vi "Initialize Digital IO.vi"(8 "error in (no error)":errorcluster, 11 "DigitalIO in":refnum<class "DigitalIO.lvclass">) -> (0 "error out":errorcluster, 3 "DigitalIO out":refnum<class "DigitalIO.lvclass">)   [LabVIEW 2018, in "DigitalIO.lvlib" / "DigitalIO.lvclass"]
uses:
  DigitalIO.lvclass
  DigitalIO.lvclass/DigitalIO.ctl
  PPLs/Configuration/Configuration.lvlibp/Configuration.lvclass
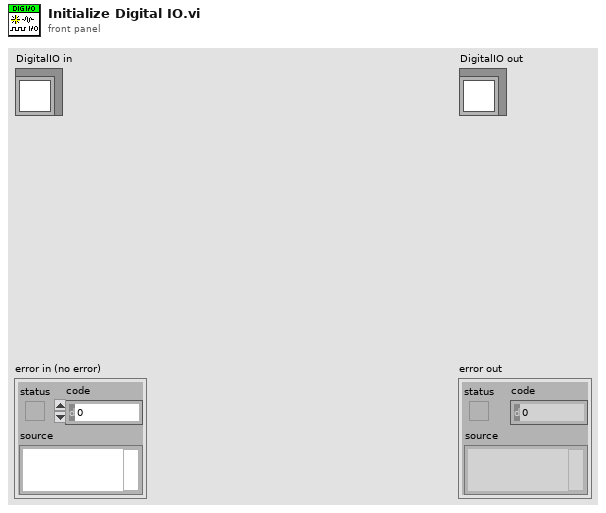
[diagram p1: front panel]
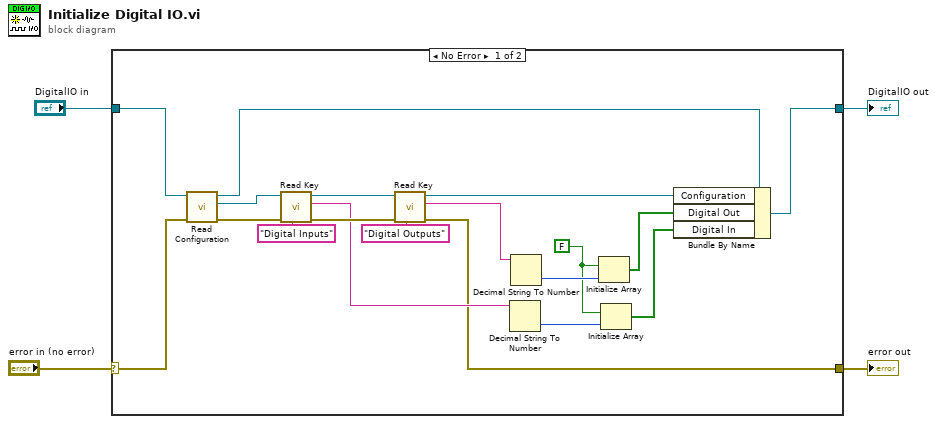
[diagram p0: block diagram]
diagram:
  n1 = case shown="No Error" "error in (no error)" {
    selector: "error in (no error)" -> [w23 w25]
    tunnel: [w5 w25] -> w1
    tunnel: [w6 w24] -> w2
    tunnel: "DigitalIO in" -> [w22 w24]
    frame No Error {
      w11 = FALSE
      n2 = call "Read Configuration.vi"("error in (no error)"=w23, "DigitalIO in"=w22) -> ("error out"=w20:errorcluster, "Configuration"=w21:refnum<class "Configuration.lvclass">, "DigitalIO out"=w10:refnum<class "DigitalIO.lvclass">)  [unwired: 7 in]
      n3 = call "Read Key.vi"("Key:"="Digital Inputs", "error in"=w20, "Configuration in"=w21) -> ("error out"=w16:errorcluster, "Value"=w15:string, "Configuration out"=w17:refnum<class "Configuration.lvclass">)  [unwired: 6 in]
      n4 = call "Read Key.vi"("Key:"="Digital Outputs", "error in"=w16, "Configuration in"=w17) -> ("error out"=w5:errorcluster, "Value"=w14:string, "Configuration out"=w9:refnum<class "Configuration.lvclass">)  [unwired: 6 in]
      n5 = Decimal String To Number(string=w15) -> (number=w12:i32)  [unwired: 2 in, 1 out]
      n6 = Decimal String To Number(string=w14) -> (number=w13:i32)  [unwired: 2 in, 1 out]
      n7 = Initialize Array(w11, w13) -> (w8:bool[])
      n8 = Initialize Array(w11, w12) -> (w7:bool[])
      n9 = Bundle By Name(cluster=w10, "Configuration"=w9, "Digital Out"=w8, "Digital In"=w7) -> (w6:refnum<class "DigitalIO.lvclass">)
    }
    frame Error {
    }
  }
  "error out" <- w1
  "DigitalIO out" <- w2
